vi "test17.2-RegisterStatusAsInterruptFromNonCSM_State.vi"(8 "error in (no error)":errorcluster, 11 "TestCase in":refnum<class "testcase-CSMBroadcast.lvclass">) -> (0 "error out":errorcluster, 3 "TestCase out":refnum<class "testcase-CSMBroadcast.lvclass">)   [LabVIEW 2017, in "testcase-CSMBroadcast.lvclass"]
uses:
  testcase-CSMBroadcast.lvclass
  src/user.lib/_NEVSTOP/Communicable State Machine(CSM)/AdvanceAPI/CSM - Broadcast Message Type.ctl
  <vilib>/addons/_JKI Toolkits/VI Tester/TestCase.llb/TestCase.lvclass
  src/user.lib/_NEVSTOP/Communicable State Machine(CSM)/Communicable State Machine.lvlib
  CSM/CSM-Testcase.lvlib
  C:/Program Files (x86)/National Instruments/LabVIEW 2017/vi.lib/addons/_JKI Toolkits/VI Tester/TestCase.llb/TestCase.lvclass
panel:
  out "output cluster":T1
  out "LoopCount":i32
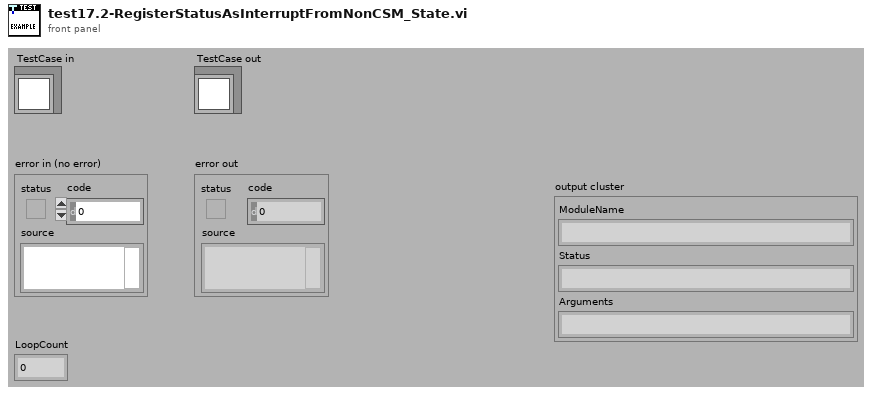
[diagram p1: front panel]
types:
  T1 = cluster{"ModuleName":string, "Status":string, "Arguments":string}
  T2 = typedef "Communicable State Machine.lvlib/CSM - Broadcast Message Type.ctl" = enum16{"<Null>", "Status", "Interrupt"}
  T3 = cluster{"Status Event":refnum<user-event>, "Interrupt Event":refnum<user-event>}
  T4 = cluster{"cluster":cluster{"ModuleName":string, "Status":string, "Arguments":string}}
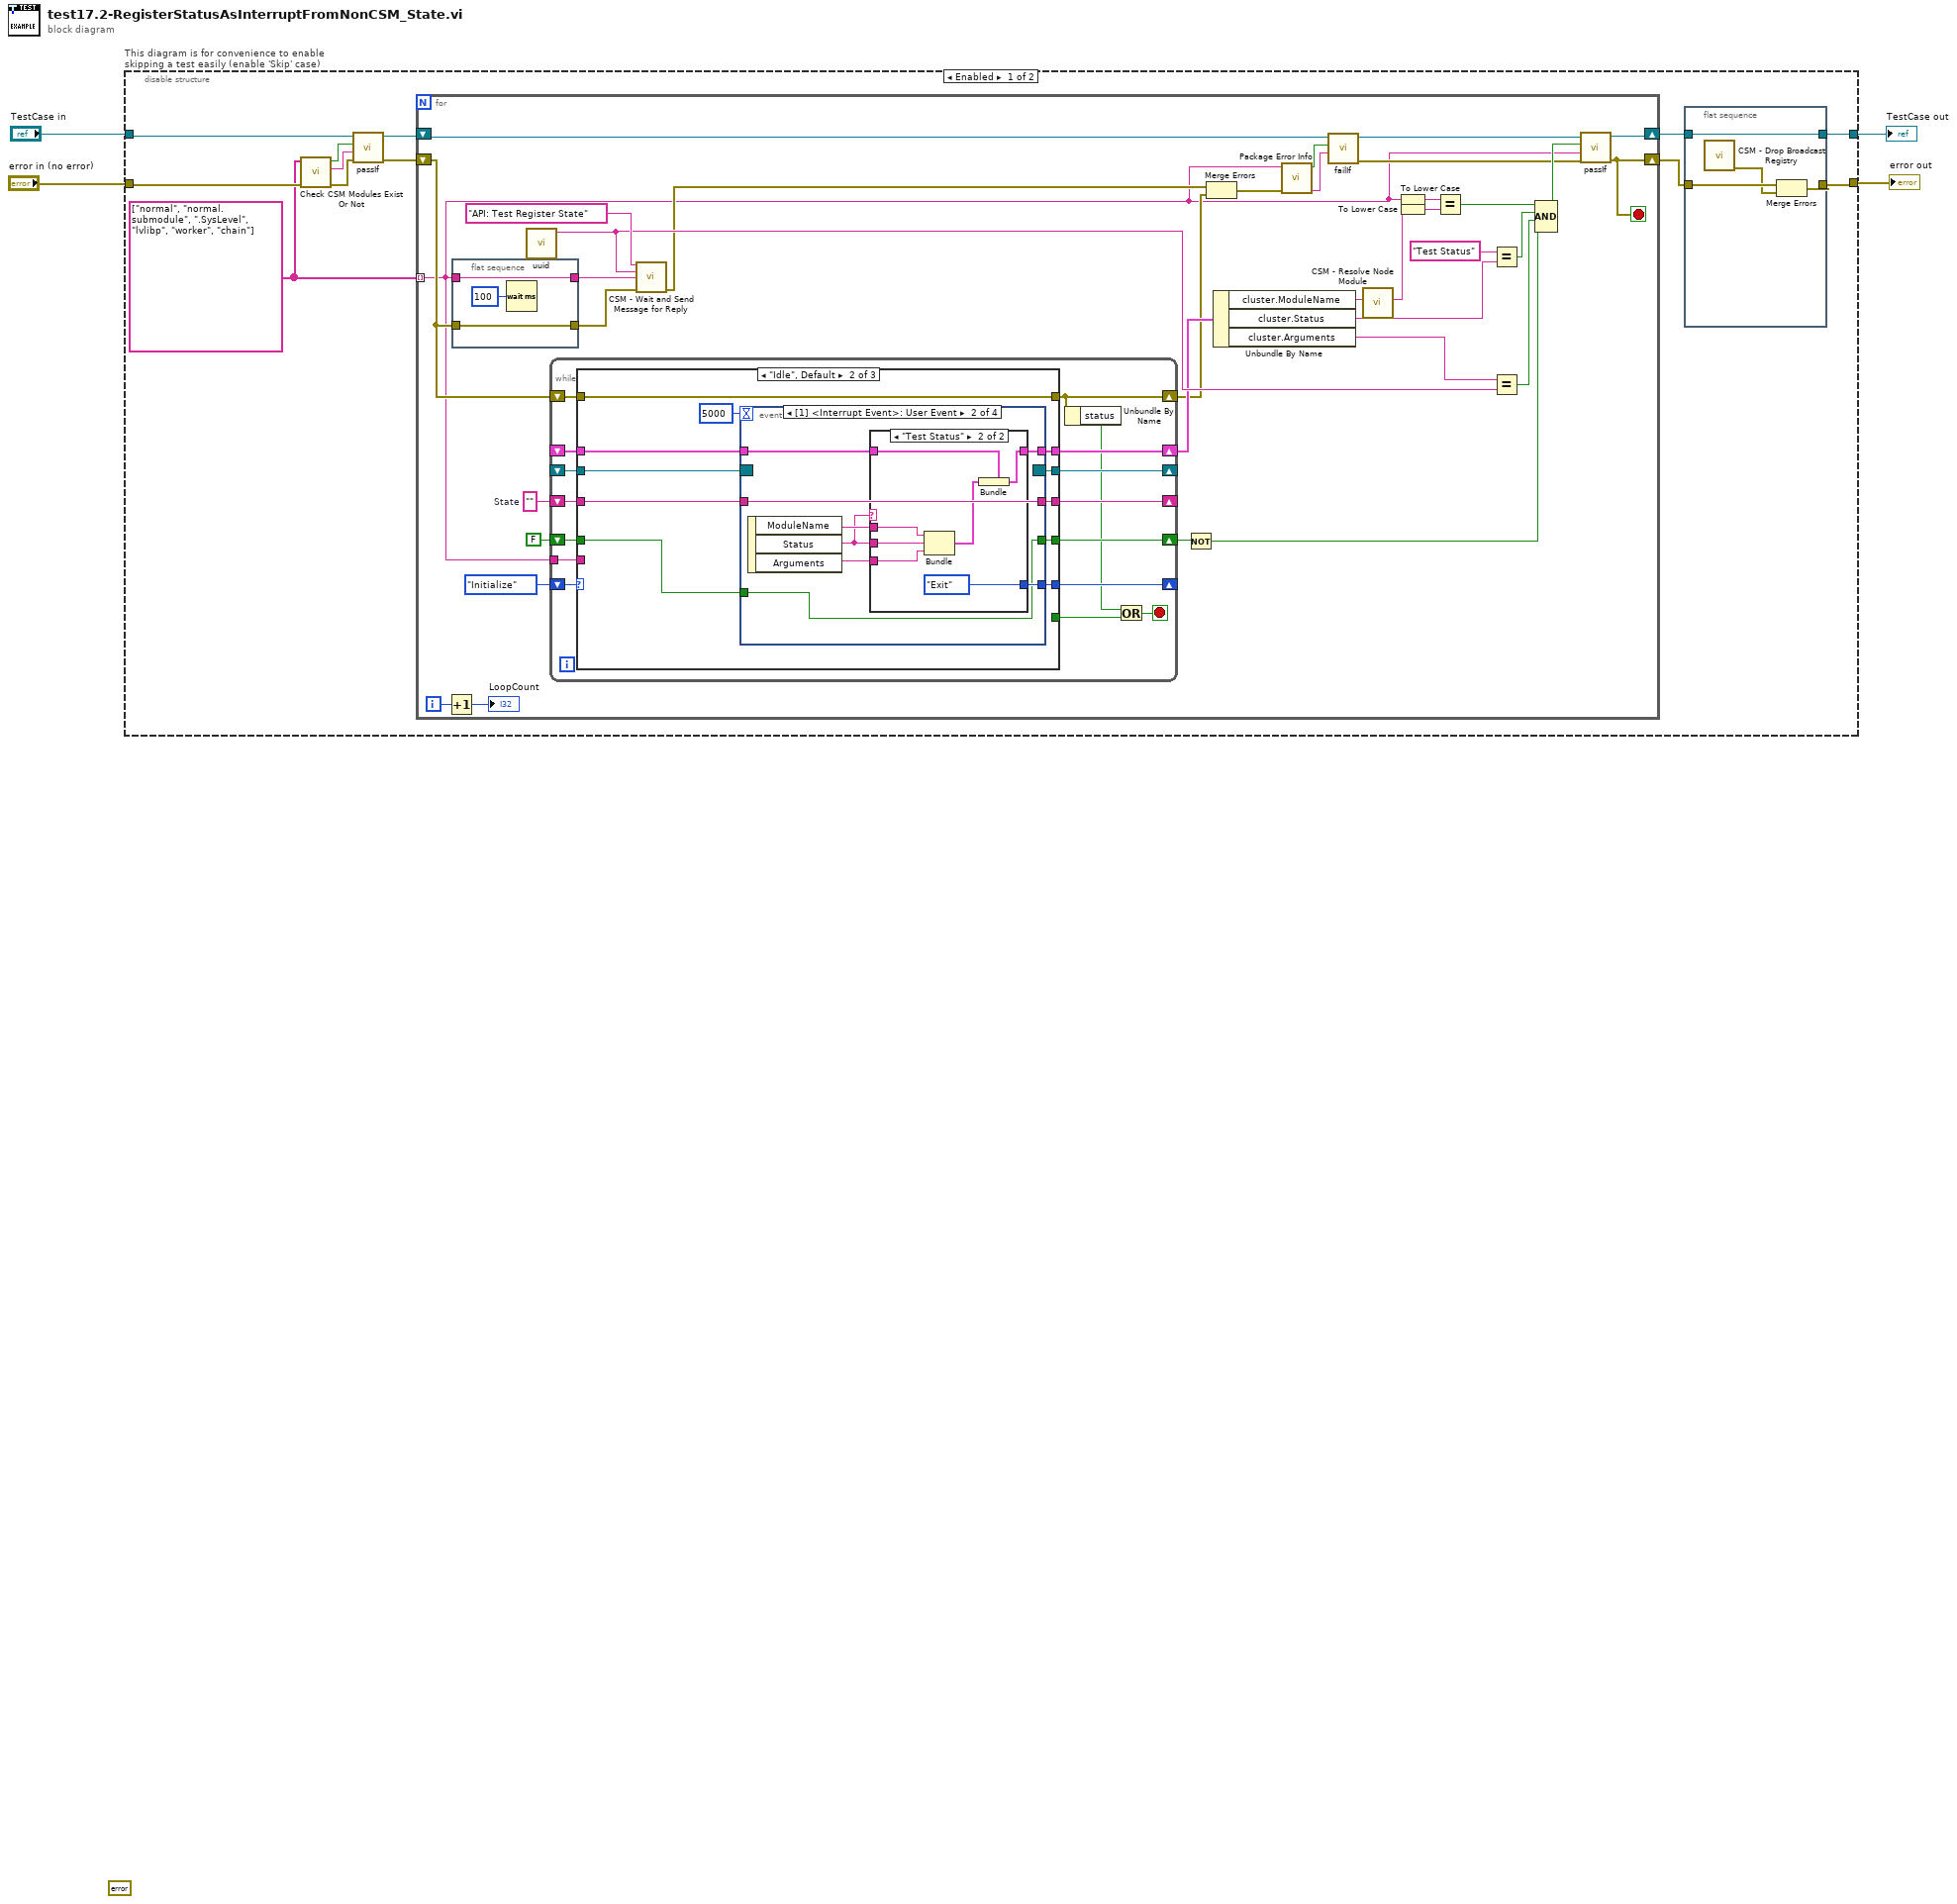
[diagram p0: block diagram]
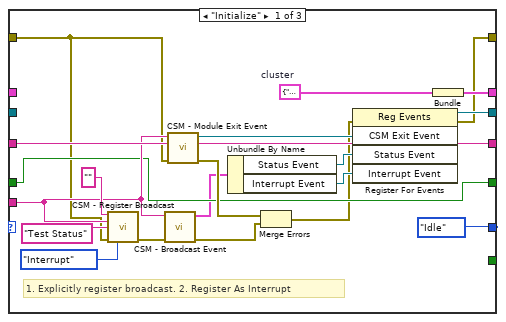
[diagram p2: hidden frame]
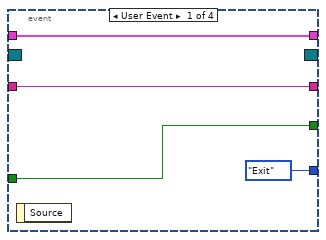
[diagram p3: hidden frame]
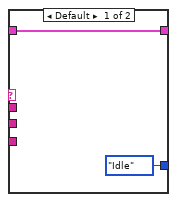
[diagram p4: hidden frame]
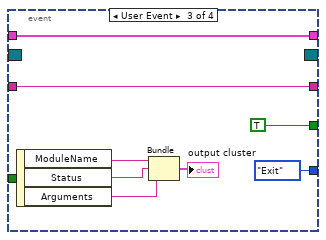
[diagram p5: hidden frame]
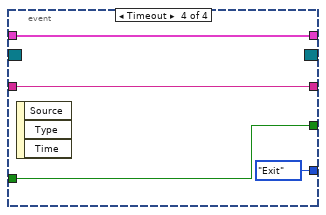
[diagram p6: hidden frame]
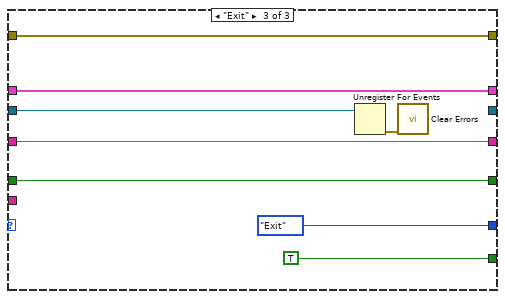
[diagram p7: hidden frame]
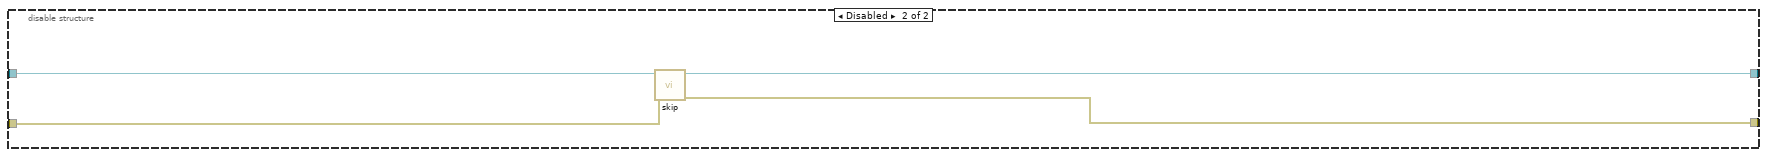
[diagram p8: hidden frame]
diagram:
  (unwired) errorcluster {"status"=FALSE, "code"=0, "source"=""} ("error out")
  n1 = disable-structure "This diagram is for convenience to enable skipping a test easily (enable 'Skip' case)" shown="Enabled" {
    disable-tunnel: "TestCase in" -> [w13 w150]
    disable-tunnel: [w7 w148] -> w2
    disable-tunnel: [w5 w149] -> w1
    disable-tunnel: "error in (no error)" -> [w11 w147]
    frame Enabled {
      w9 = string[] ["normal", "normal.submodule", ".SysLevel", "lvlibp", "worker", "chain"]
      n2 = call "Check CSM Modules Exist Or Not.vi"("error in"=w11, "CSM names in"=w9) -> ("error out"=w14:errorcluster, "Debug string"=w15:string, "All Modules Exist?"=w16:bool)  [unwired: 7 in]
      n3 = call-dynamic "passIf.vi"("error in (no error)"=w14, "message (\"\")"=w15, "pass"=w16, "TestCase in"=w13) -> ("error out"=w10:errorcluster, "TestCase out"=w12:refnum<class "testcase-CSMBroadcast.lvclass">)  [unwired: 6 in]
      n4 = for {
        shift-right: [w47] -> w8
        shift-left: w12 -> [w27]
        tunnel: w9 -> [w21] mode=indexing
        shift-right: [w40] -> w6
        shift-left: w10 -> [w30]
        i -> [w42]
        stop <- w40 stop-if-true
        w54 = ""  # State
        n5 = Increment(x=w42) -> (x+1=→"LoopCount":i32)
        n6 = flat-sequence {
          tunnel: w21 -> [w58]
          tunnel: [w58] -> w52
          tunnel: [w56] -> w31
          tunnel: w30 -> [w56]
          frame #0 {
            n7 = Wait (ms)(milliseconds to wait=u32 100) -> ()  [unwired: 1 out]
          }
        }
        n8 = call "uuid.vi"() -> ("UUID"=w49:string)  [unwired: 11 in]
        n9 = while {
          shift-right: [w73] -> _
          shift-left: enum16{"Idle", "Initialize", "Exit"}."Initialize" -> [w74]
          shift-right: [w71] -> _
          shift-left: w54 -> [w72]
          shift-right: [w70] -> _
          shift-left: _ -> [w69]
          shift-right: [w68] -> w39
          shift-left: _ -> [w67]
          tunnel: w21 -> [w66]
          shift-right: [w65] -> w34
          shift-left: FALSE -> [w64]
          shift-right: [w60] -> w23
          shift-left: w30 -> [w63]
          stop <- w62 stop-if-true
          n10 = case shown="\"Idle\", Default" w74 {
            tunnel: [enum16{"Idle", "Initialize", "Exit"}."Idle" w105 enum16{"Idle", "Initialize", "Exit"}."Exit"] -> w73
            tunnel: [_ _ TRUE] -> w61
            tunnel: w72 -> [w93 w103 w144]
            tunnel: [w93 w104 w144] -> w71
            tunnel: [w91 w101 _] -> w70
            tunnel: w69 -> [_ w102 w143]
            tunnel: [w90 w99 w141] -> w68
            tunnel: w67 -> [_ w100 w141]
            tunnel: w66 -> [w83 _ _]
            tunnel: [w80 w97 w140] -> w65
            tunnel: w64 -> [w80 w96 w140]
            tunnel: w63 -> [w77 w95 w139]
            tunnel: [w75 w95 w139] -> w60
            frame "Initialize" {
              w89 = T1 {"ModuleName"="", "Status"="", "Arguments"=""}  # cluster
              # "1. Explicitly register broadcast. 2. Register As Interrupt"
              n11 = call "CSM - Register Broadcast.vi"("CSM Name(Empty for Broadcast Event)"="", "Source CSM Name (* as Default)"=w83, "Trigger"="Test Status" ("State"), "Error In"=w77, "Priority (No Change)"=CSM_-_Broadcast_Message_Type."Interrupt" ("Priority(No Change)")) -> ("error out"=w85:errorcluster)  [unwired: 9 in, 1 out]
              n12 = call "CSM - Broadcast Event.vi"("Error In"=w85, "CSM Module"=w83) -> ("error out"=w87:errorcluster, "Broadcast Event"=w79:T3)  [unwired: 7 in, 1 out]
              n13 = call "CSM - Module Exit Event.vi"("Error In"=w77, "Name (\"\" to Use UUID) In"=w83) -> ("error out"=w88:errorcluster, "CSM Exit Event"=w92:refnum<user-event>)  [unwired: 7 in, 1 out]
              n14 = Unbundle By Name(w79) -> ("Status Event"=w82:refnum<user-event>, "Interrupt Event"=w81:refnum<user-event>)
              n15 = Merge Errors(w88, w87) -> (w76:errorcluster)
              n16 = register-events(error in=w76, w92, w82, w81) -> (reference out=w91:refnum<event-registration>, error out=w75:errorcluster)  [unwired: 1 in]
              n17 = Bundle("cluster"=w89) -> (w90:T4)  [unwired: 1 in]
            }
            frame "Idle", Default {
              n18 = event shown="[1] <Interrupt Event>: User Event" {
                selector: w102 -> [_ _ _ _]
                dyn-events: [_ _ _ _] -> w101
                timeout: 5000 -> [_ _ _ _]
                tunnel: [enum16{"Idle", "Initialize", "Exit"}."Exit" w116 enum16{"Idle", "Initialize", "Exit"}."Exit" enum16{"Idle", "Initialize", "Exit"}."Exit"] -> w105
                tunnel: w103 -> [w109 w117 w134 w138]
                tunnel: [w109 w117 w134 w138] -> w104
                tunnel: w100 -> [w107 w113 w133 w137]
                tunnel: [w107 w112 w133 w137] -> w99
                tunnel: [w106 w110 TRUE w135] -> w97
                tunnel: w96 -> [w106 w110 _ w135]
                event User Event {
                  n19 = event-data() -> ()  [unwired: 1 in, 1 out]
                }
                event User Event {
                  n20 = event-data() -> ("ModuleName"=w115:string, "Status"=w111:string, "Arguments"=w114:string)  [unwired: 1 in]
                  n21 = case shown="\"Test Status\"" w111 {
                    tunnel: [enum16{"Idle", "Initialize", "Exit"}."Idle" enum16{"Idle", "Initialize", "Exit"}."Exit"] -> w116
                    tunnel: w115 -> [_ w125]
                    tunnel: w111 -> [_ w124]
                    tunnel: w114 -> [_ w123]
                    tunnel: w113 -> [w119 w122]
                    tunnel: [w119 w120] -> w112
                    frame Default {
                    }
                    frame "Test Status" {
                      n22 = Bundle("ModuleName"=w125, "Status"=w124, "Arguments"=w123) -> (w121:T1)  [unwired: 1 in]
                      n23 = Bundle(cluster=w122, "cluster"=w121) -> (w120:T4)
                    }
                  }
                }
                event User Event {
                  n24 = event-data() -> ("ModuleName"=w130:string, "Status"=w129:string, "Arguments"=w128:string)  [unwired: 1 in]
                  n25 = Bundle("ModuleName"=w130, "Status"=w129, "Arguments"=w128) -> (→"output cluster":T1)  [unwired: 1 in]
                }
                event Timeout {
                  n26 = event-data() -> ()  [unwired: 1 in, 3 out]
                }
              }
            }
            frame "Exit" {
              n27 = Unregister For Events(event registration refnum=w143) -> (error out=w142:errorcluster)  [unwired: 1 in]
              n28 = call <vilib>:"Clear Errors.vi"("error in (no error)"=w142) -> ()  [unwired: 5 in, 2 out]
            }
          }
          n29 = Unbundle By Name(w60) -> ("status"=w59:bool)
          n30 = Or(x=w59, y=w61) -> (x .or. y?=w62:bool)
        }
        n31 = call "CSM - Wait and Send Message for Reply.vi"("State"="API: Test Register State", "Arguments (\"\")"=w49, "Target Module"=w52, "Error In (No Error)"=w31) -> ("error out"=w24:errorcluster)  [unwired: 8 in, 3 out]
        n32 = Not(x=w34) -> (.not. x?=w33:bool)
        n33 = Merge Errors(w24, w23) -> (w22:errorcluster)
        n34 = Unbundle By Name(w39) -> ("cluster.ModuleName"=w37:string, "cluster.Status"=w50:string, "cluster.Arguments"=w48:string)
        n35 = call "Package Error Info.vi"("error in"=w22, "String in"=w21) -> ("packed error info out"=w28:string, "error status"=w29:bool)  [unwired: 8 in]
        n36 = call-dynamic "failIf.vi"("message (\"\")"=w28, "fail"=w29, "TestCase in"=w27) -> ("error out"=w25:errorcluster, "TestCase out"=w26:refnum<class "testcase-CSMBroadcast.lvclass">)  [unwired: 7 in]
        n37 = call "CSM - Resolve Node Module.vi"("Node Name"=w37) -> ("CSM Module Name"=w35:string)  [unwired: 10 in]
        n38 = To Lower Case(string=w21) -> (all lower case string=w38:string)
        n39 = To Lower Case(string=w35) -> (all lower case string=w36:string)
        n40 = Equal?(x=w38, y=w36) -> (x = y?=w46:bool)
        n41 = Equal?(x="Test Status" ("State"), y=w50) -> (x = y?=w45:bool)
        n42 = Equal?(x=w48, y=w49) -> (x = y?=w44:bool)
        n43 = Compound Arithmetic op=AND(w46, w45, w44, w33) -> (w43:bool)
        n44 = call-dynamic "passIf.vi"("error in (no error)"=w25, "message (\"\")"=w21, "pass"=w43, "TestCase in"=w26) -> ("error out"=w40:errorcluster, "TestCase out"=w47:refnum<class "testcase-CSMBroadcast.lvclass">)  [unwired: 6 in]
      }
      n45 = flat-sequence {
        tunnel: w6 -> [w20]
        tunnel: [w19] -> w5
        tunnel: w8 -> [w17]
        tunnel: [w17] -> w7
        frame #0 {
          n46 = call "CSM - Drop Broadcast Registry.vi"() -> ("error out"=w18:errorcluster)  [unwired: 15 in]
          n47 = Merge Errors(w20, w18) -> (w19:errorcluster)
        }
      }
    }
    frame Disabled {
      # "skip test result while test is under development"
      n48 = call <vilib>:"skip.vi"("error in (no error)"=w147, "TestCase in"=w150) -> ("error out"=w149:errorcluster, "TestCase out"=w148:refnum<class "testcase-CSMBroadcast.lvclass">)  [unwired: 8 in]
    }
  }
  "error out" <- w1
  "TestCase out" <- w2
